vi "API Feed Motor START.vi"() -> (2 "feedmotorstart return value":bool)   [LabVIEW 2011, in "API DYM.lvlib"]
uses:
  API DYM.lvlib
  DyMechnicalPlatform.dll
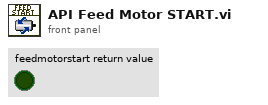
[diagram p1: front panel]
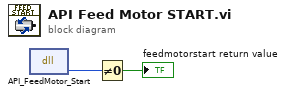
[diagram p0: block diagram]
diagram:
  n1 = dll-call lib="PTH1Xabs D可重构机电平台项目DemoLabViewDYSYSAPIDyMechnicalPlatform.dll" fn="API_FeedMotor_Start"() -> ("返回类型"=w2:i32)  [unwired: 3 in, 2 out]
  n2 = Not Equal To 0?(x=w2) -> (x != 0?=→"feedmotorstart return value":bool)
